vi "L18.vi"() -> ()   [LabVIEW 2012]
panel:
  out "Waveform Graph":i32[](graph)
  out "subarray":i32[](array[numeric])
  out "max value":i32
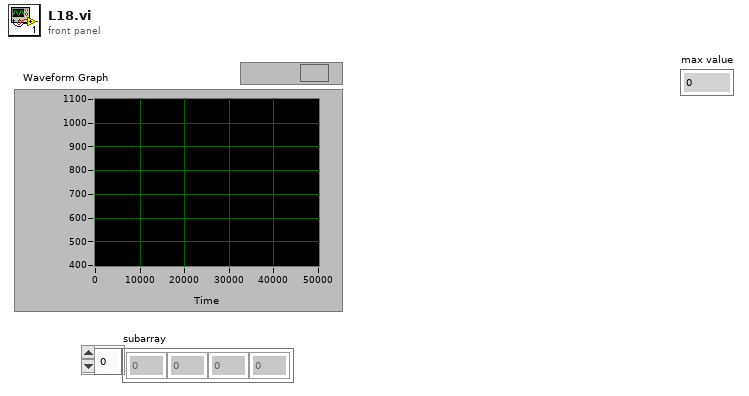
[diagram p1: front panel]
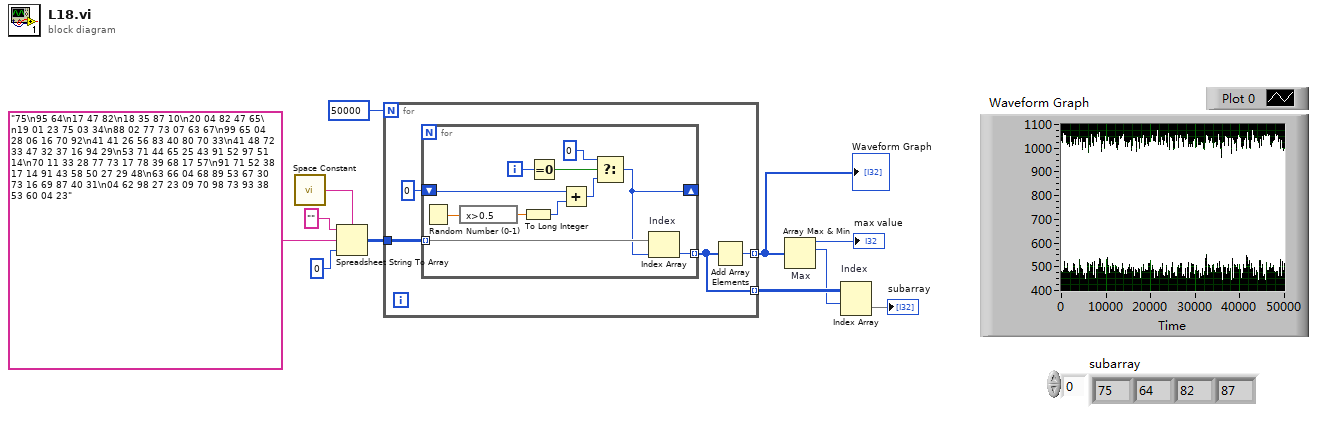
[diagram p0: block diagram]
diagram:
  n1 = call <vilib>:"Space Constant.vi"() -> ("String"=w11:string)
  n2 = Spreadsheet String To Array(delimiter (Tab)=w11, format string="", spreadsheet string="75\n95 64\n17 47 82\n18 35 87 10\n20 04 82 47 65\n19 01 23 75 03 34\n88 02 77 73 07 63 67\n99 65 04 28 06 16 70 92\n41 41 26 56 83 40 80 70 33\n41 48 72 33 47 32 37 16 94 29\n53 71 44 65 25 43 91 52 97 51 14\n70 11 33 28 77 73 17 78 39 68 17 57\n91 71 52 38 17 14 91 43 58 50 27 29 48\n63 66 04 68 89 53 67 30 73 16 69 87 40 31\n04 62 98 27 23 09 70 98 73 93 38 53 60 04 23" ("format string"), array type (2D Dbl)=0) -> (array=w8:i32[][])
  n3 = for {
    N: 50000 -> [_]
    tunnel: w8 -> [w15]
    tunnel: [w13] -> w2 mode=indexing
    tunnel: [w12] -> w5 mode=indexing
    n4 = for {
      tunnel: w15 -> [w26] mode=indexing
      shift-right: [w16] -> _
      shift-left: 0 -> [w25]
      tunnel: [w24] -> w12 mode=indexing
      i -> [w20]
      n5 = Random Number (0-1)() -> (number: 0 to 1=w23:dbl)
      n6 = expression code="x>0.5"(w23) -> (w22:dbl)
      n7 = To Long Integer(number=w22) -> (32bit integer=w21:i32)
      n8 = Equal To 0?(x=w20) -> (x = 0?=w18:bool)
      n9 = Add(x=w25, y=w21) -> (x+y=w19:i32)
      n10 = Select(t=0, s=w18, f=w19) -> (s? t:f=w16:i32)
      n11 = Index Array "Index"(array=w26, index=w16) -> (element=w24:i32)
    }
    n12 = Add Array Elements(numeric array=w12) -> (sum=w13:i32)
  }
  "Waveform Graph" <- w2
  n13 = Array Max & Min "Max"(array=w2) -> (max value=→"max value":i32, max index (indices)=w4:i32)  [unwired: 2 out]
  n14 = Index Array "Index"(array=w5, index (row)=w4) -> (element=→"subarray":i32[])  [unwired: 1 in]
